vi "GetNet-Client Send Message.vi"(8 "error in":errorcluster, 10 "Message Data":variant, 11 "Data Cluster in":T1) -> (0 "error out":errorcluster, 2 "Return Message Data":variant, 3 "Data Cluster out":T1)   [LabVIEW 2022 SP3, in "GenNet-Client.lvlib"]
doc: "Checks the TCP network connection, writes the message out, waits for the reply from the server and reports the response and/or an error to the parent (caller).\n\n____\nHAMPEL SOFTWARE ENGINEERING v3.8.0 (2023-12-18 14:41)"
uses:
  GenNet-Client.lvlib
  Module Data--cluster.ctl
  GenNet Protocols/GenNet Protocol.lvclass
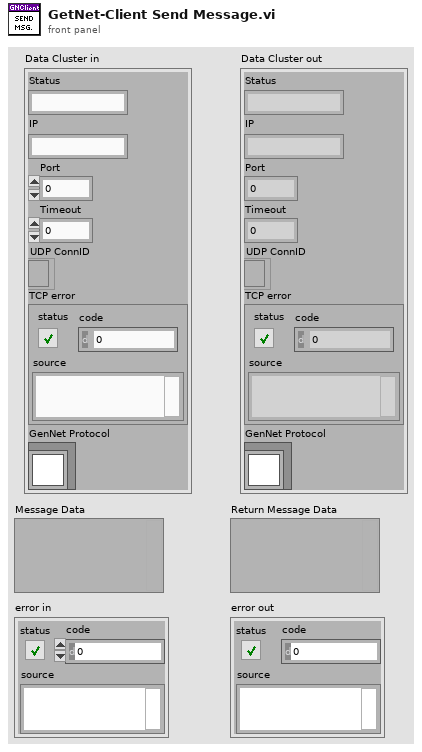
[diagram p1: front panel]
types:
  T1 = typedef "GenNet-Client.lvlib/Module Data--cluster.ctl" = cluster{"Status":string, "IP":string, "Port":u16, "Timeout":i32, "UDP ConnID":refnum<k16>, "TCP error":errorcluster, "GenNet Protocol":refnum<class "GenNet Protocol.lvclass">}
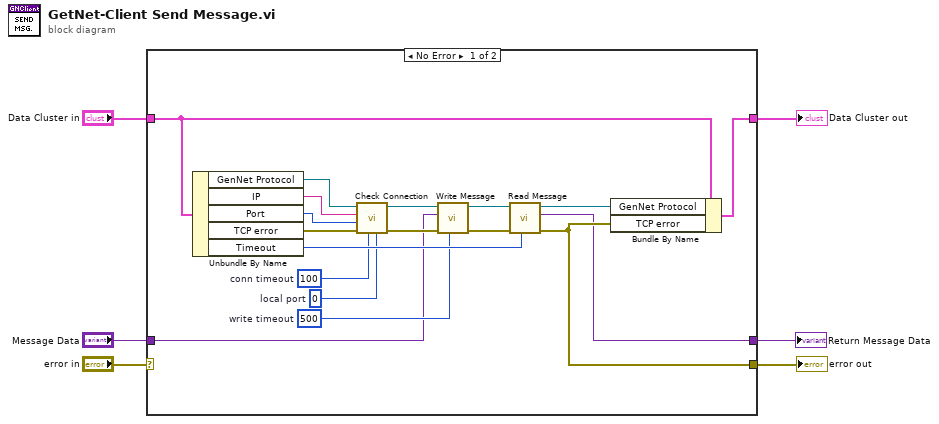
[diagram p0: block diagram]
diagram:
  n1 = case shown="No Error" "error in" {
    selector: "error in" -> [_ w26]
    tunnel: [w23 w26] -> w6
    tunnel: [w10 w25] -> w5
    tunnel: "Data Cluster in" -> [w9 w25]
    tunnel: "Message Data" -> [w8 _]
    tunnel: [w7 _] -> w1
    frame No Error {
      w21 = 500  # write timeout
      w20 = u16 0  # local port
      w19 = 100  # conn timeout
      n2 = Unbundle By Name(w9) -> ("GenNet Protocol"=w14:refnum<class "GenNet Protocol.lvclass">, "IP"=w17:string, "Port"=w18:u16, "TCP error"=w24:errorcluster, "Timeout"=w22:i32)
      n3 = call-dynamic "Check Connection.vi"("local port (0)"=w20, "timeout [ms]"=w19, "error in (no error)"=w24, "remote port"=w18, "ip address"=w17, "GenNet Protocol in"=w14) -> ("error out"=w16:errorcluster, "GenNet Protocol out"=w15:refnum<class "GenNet Protocol.lvclass">)  [unwired: 4 in]
      n4 = call-dynamic "Write Message.vi"("timeout ms (25000)"=w21, "error in (no error)"=w16, "Message"=w8, "GenNet Protocol in"=w15) -> ("error out"=w13:errorcluster, "GenNet Protocol out"=w11:refnum<class "GenNet Protocol.lvclass">)  [unwired: 6 in]
      n5 = call-dynamic "Read Message.vi"("timeout ms (25000)"=w22, "error in (no error)"=w13, "GenNet Protocol in"=w11) -> ("error out"=w23:errorcluster, "Message"=w7:variant, "GenNet Protocol out"=w12:refnum<class "GenNet Protocol.lvclass">)  [unwired: 6 in]
      n6 = Bundle By Name(cluster=w9, "GenNet Protocol"=w12, "TCP error"=w23) -> (w10:T1)
    }
    frame Error {
    }
  }
  "error out" <- w6
  "Data Cluster out" <- w5
  "Return Message Data" <- w1
